vi "__vna_read_save_takeAwayBackground.vi"() -> ()   [LabVIEW 2013]
panel:
  in  "Take Away Background?":bool=TRUE
  in  "Gain":cluster{dbl[], dbl[]}(graph)={array[1001 elements], array[1001 elements]}
  in  "Tab Control 2":enum32{"Page 1", "Page 2"}(tab)
  in  "Power dBm":dbl=-20.0 caption="Power, dBm" format="%#.3f"
  in  "Start Freq (Hz)":dbl=100000.0 min=100000.0 max=20000000000.0 format="%^#.6e"
  in  "Stop Freq":dbl=200000000.0 caption="Stop Freq (Hz):" format="%^#.3e"
  in  "Bandwidth:":dbl=100.0 caption="Bandwidth (1 to 1e6 Hz):" format="%#.3f"
  in  "Points:":i32=1001
  in  "Tab Control":enum32{"Page 1"}(tab)
  in  "Boolean":bool
  in  "Name":string="data_labview_vna_(2)gain_len"
  out "Phase":cluster{dbl[], dbl[]}(graph)
  out "Gain":cluster{dbl[], dbl[]}(graph)
  # "BACKGROUND"
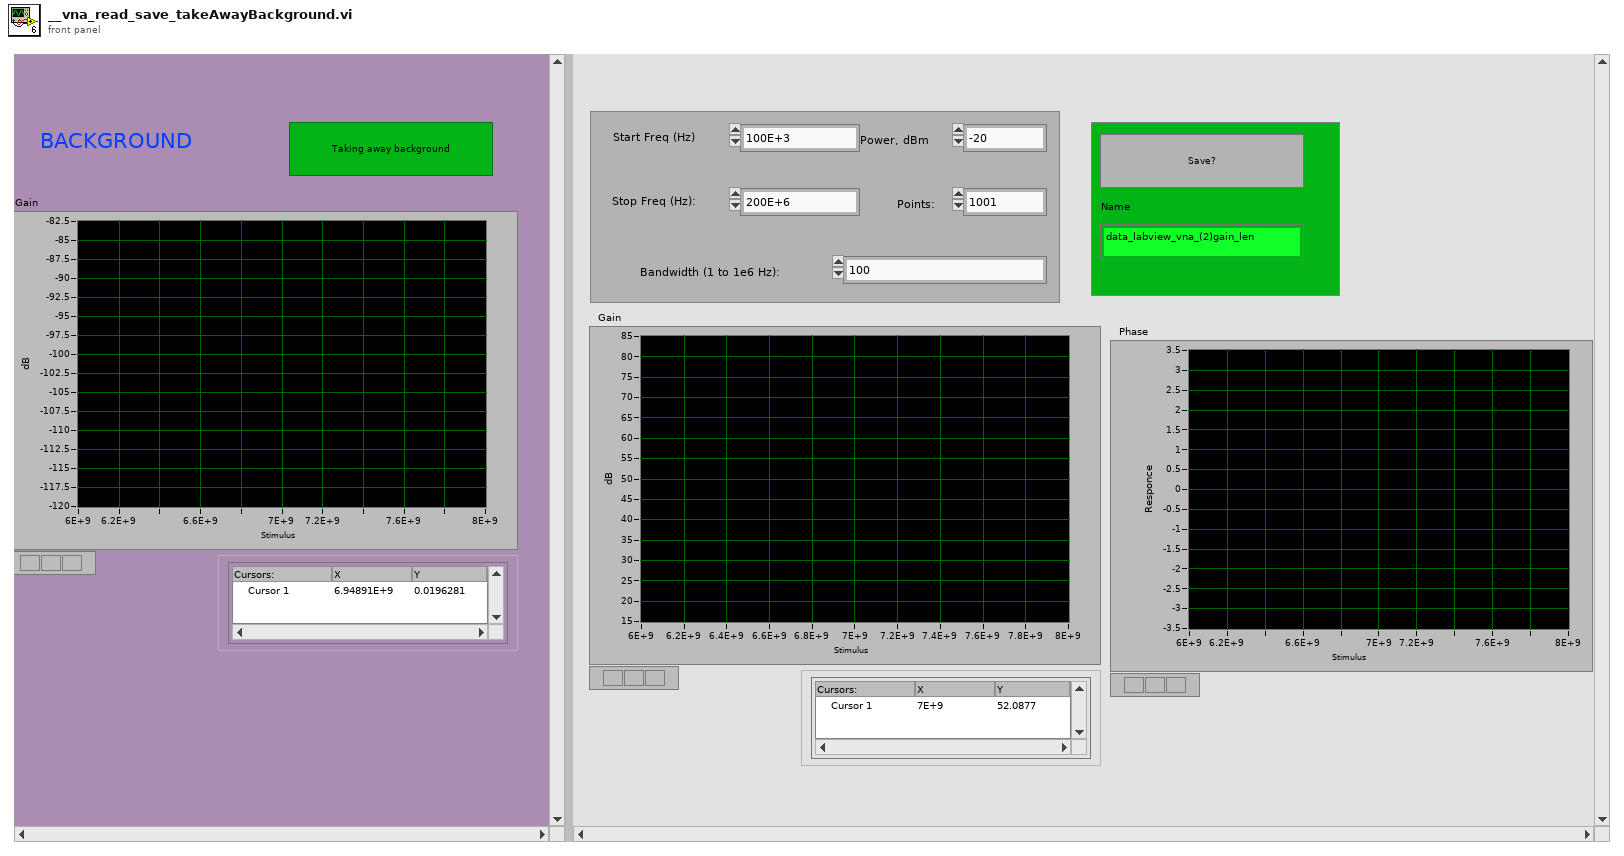
[diagram p1: front panel]
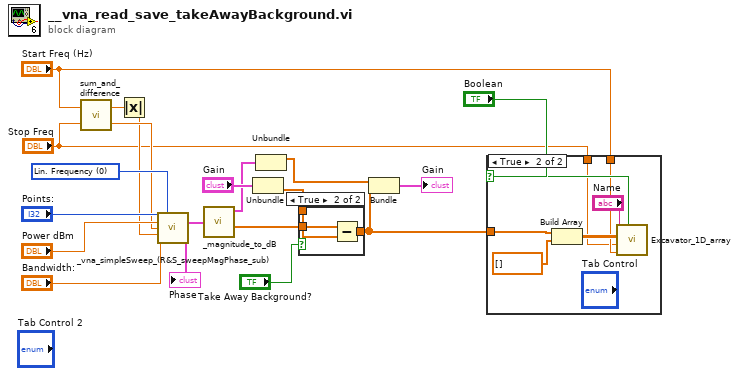
[diagram p0: block diagram]
diagram:
  w18 = 0 items=["Lin. Frequency", "Log. Frequency", "Segmented Frequency", "Power", "CW Mode", "Time"] ("Sweep Type")
  n1 = call "sum_and_difference.vi"("Begin"="Stop Freq", "End"="Start Freq (Hz)") -> ("Mid Point"=w12:dbl, "Difference (abs)"=w13:dbl)
  n2 = Absolute Value(x=w13) -> (abs(x)=w11:dbl)
  n3 = call "_vna_simpleSweep_(R&S_sweepMagPhase_sub).vi"("Sweep Type"=w18, "Points:"="Points:", "Power dBm"="Power dBm", "Center Freq:"=w12, "Span Freq:"=w11, "Bandwidth:"="Bandwidth:") -> ("Lin Mag"=w14:cluster{dbl[], dbl[]}, "Phase"=→"Phase":cluster{dbl[], dbl[]})  [unwired: 8 in]
  n4 = call "_magnitude_to_dB.vi"("Lin Mag in"=w14) -> ("Cluster"=w2:cluster{dbl[], dbl[]}, "dB"=w6:dbl[])  [unwired: 2 out]
  n5 = Unbundle("Gain") -> (w8:dbl[])  [unwired: 1 out]
  n6 = Unbundle(w2) -> (w1:dbl[])  [unwired: 1 out]
  n7 = case shown="True" "Take Away Background?" {
    tunnel: w8 -> [_ w24]
    tunnel: w6 -> [w21 w23]
    tunnel: [w21 w22] -> w5
    frame False {
    }
    frame True {
      n8 = Subtract(x=w23, y=w24) -> (x-y=w22:dbl[])
    }
  }
  n9 = Bundle(w1, "dB"=w5) -> (→"Gain":cluster{dbl[], "dB":dbl[]})  [unwired: 1 in]
  n10 = case shown="True" "Boolean" {
    selector: "Boolean" -> [_ w28]
    tunnel: w5 -> [_ w27]
    tunnel: "Start Freq (Hz)" -> [_ w26]
    tunnel: "Stop Freq" -> [_ w25]
    frame False {
    }
    frame True {
      n11 = Build Array(w27, dbl[] [] ("element")) -> (w30:dbl[][])
      n12 = call "Excavator_1D_array.vi"("Name"="Name", "Array"=w30, "x_max"=w25, "x_min"=w26, "Save?"=w28) -> ()  [unwired: 1 out]
    }
  }
